vi "Get DI param from PGserver.vi"(6 "conninfo":T1={"host"="localhost", "port"="5432", "client_encoding"="WIN1251", "dbname"="data", "user"="postgres", "password"=""}, 7 "KFM":string[](array[string]), 8 "error in (no error)":errorcluster, 9 "DIParamColumns":string[](array[string])=["invert", "time_const", "module_fcode_full", "control_channel_num", "ip_adress", "fcode", "fcodef", "fcode_full", "fname"], 10 "DIParamTable":string="fd_3", 11 "DI_fcode_full":string[](array[string])) -> (0 "error out":errorcluster, 2 "Names table":string[][](array[string]), 3 "DIParameters table":dbl[][](array[numeric]))   [LabVIEW 2019, in "Inputs.lvlib"]
uses:
  Inputs.lvlib
  Database/ctl/Coninfo.ctl
  Ctl/DIParamColumns.ctl
  Database/PostgreSQL2LabVIEW/libpqlv/src/PQfinish.vi
  Database/PostgreSQL2LabVIEW/libpqlv/src/PQconnectdb.vi
  Database/PostgreSQL2LabVIEW/libpqlv/src/PQerrorMessage.vi
  Database/PostgreSQL2LabVIEW/libpqlv/src/PQstatus.vi
  <vilib>/dlg_ctls.llb/Space Constant.vi
  Database/Progress.vi
  Database/PostgreSQL2LabVIEW/libpqUtility/libpqutility.lvlib
  Database/PostgreSQL.lvlib
  Database/PostgreSQL2LabVIEW/libpqUtility64/libpqutility64.lvlib
panel:
  out "PQStatus":T2(ring)
  # "fcode_full"
  # "fname"
  # "time_const"
  # "ip_adress"
  # "fcodef"
  # "control_channel_num"
  # "instrument_offset"
  # "module_num"
  # "fcode"
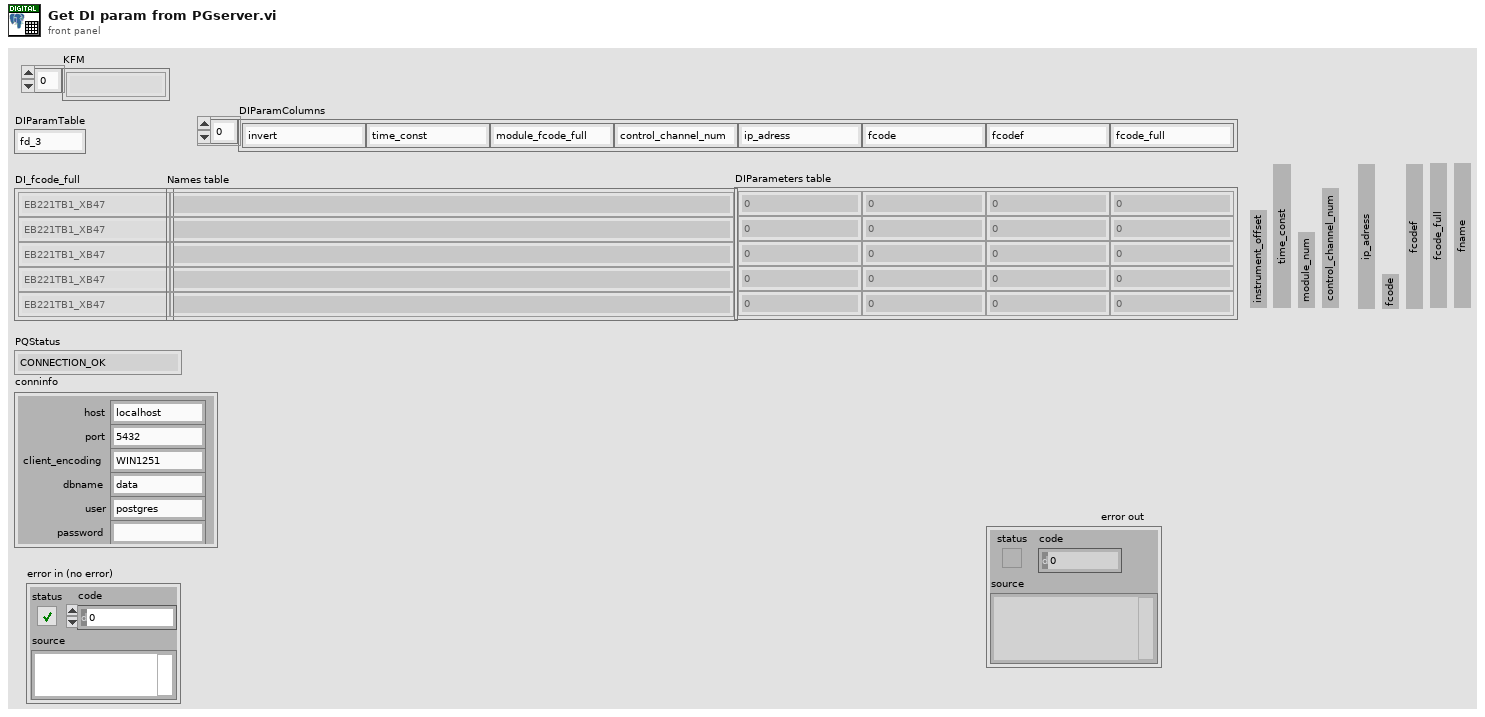
[diagram p1: front panel]
types:
  T1 = typedef "PostgreSQL.lvlib/Coninfo.ctl" = cluster{"host":string, "port":string, "client_encoding":string, "dbname":string, "user":string, "password":string}
  T2 = enum16{"CONNECTION_OK", "CONNECTION_BAD", "CONNECTION_STARTED", "CONNECTION_MADE", "CONNECTION_AWAITING_RESPONSE", "CONNECTION_AUTH_OK", "CONNECTION_SETENV", "CONNECTION_SSL_STARTUP", "CONNECTION_NEEDED"}
  T3 = typedef "Inputs.lvlib/DIParamColumns.ctl" = enum16{"invert", "time_const", "module_fcode_full", "control_channel_num", "ip_adress", "fcode", "fcodef", "fcode_full", "fname"}
  T4 = enum32{"CONNECTION_OK", "CONNECTION_BAD", "CONNECTION_STARTED", "CONNECTION_MADE", "CONNECTION_AWAITING_RESPONSE", "CONNECTION_AUTH_OK", "CONNECTION_SETENV", "CONNECTION_SSL_STARTUP", "CONNECTION_NEEDED"}
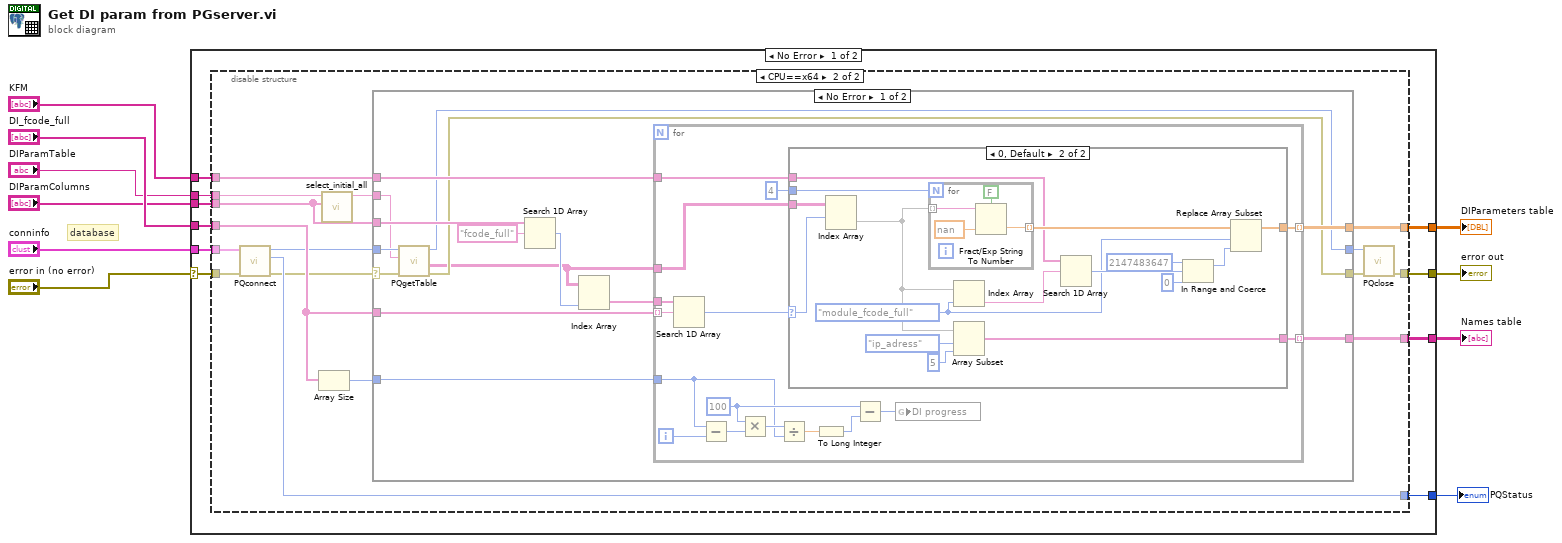
[diagram p0: block diagram]
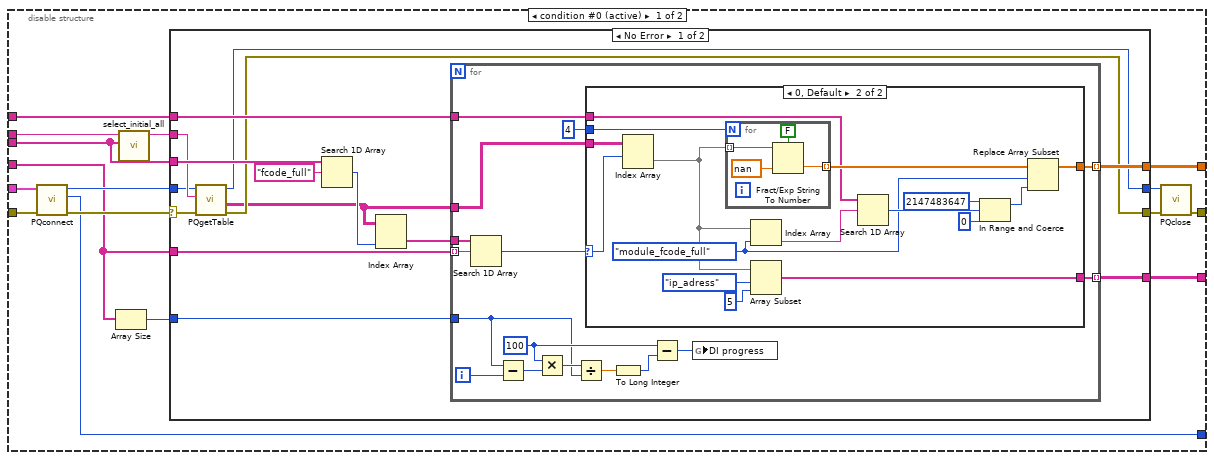
[diagram p2: hidden frame]
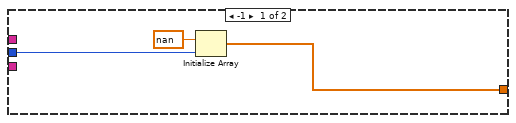
[diagram p3: hidden frame]
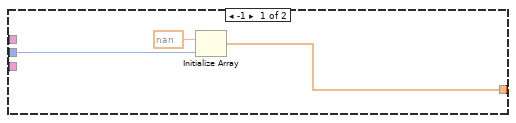
[diagram p5: hidden frame]
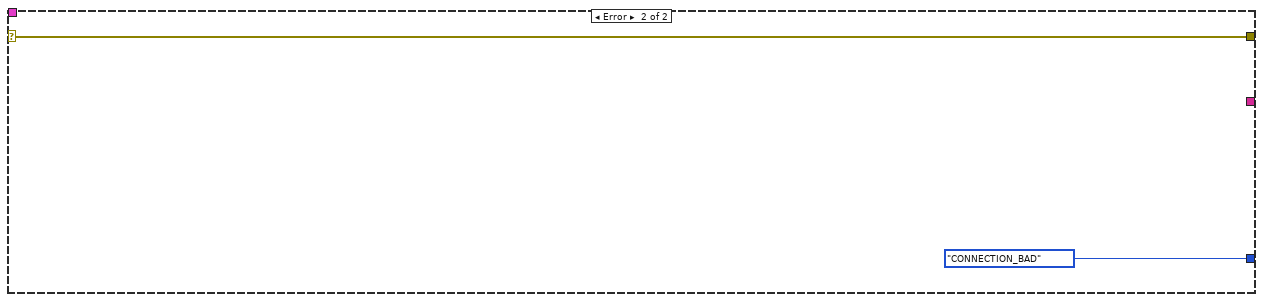
[diagram p7: hidden frame]
diagram:
  # "database"
  n1 = case shown="No Error" "error in (no error)" {
    selector: "error in (no error)" -> [w15 w166]
    tunnel: "DI_fcode_full" -> [w17 _]
    tunnel: "DIParamTable" -> [w19 _]
    tunnel: "DIParamColumns" -> [w18 _]
    tunnel: [w14 _] -> w7
    tunnel: [w13 w166] -> w6
    tunnel: [w12 _] -> w5
    tunnel: "conninfo" -> [w16 _]
    tunnel: "KFM" -> [w20 _]
    tunnel: [w11 T4."CONNECTION_BAD" ("PQStatus")] -> w1
    frame No Error {
      n2 = disable-structure shown="CPU==x64" {
        disable-tunnel: [w24 w99] -> w13
        disable-tunnel: [w29 w101] -> w14
        disable-tunnel: [w28 w102] -> w12
        disable-tunnel: w18 -> [w21 w104]
        disable-tunnel: w16 -> [w33 w97]
        disable-tunnel: w19 -> [w23 w105]
        disable-tunnel: w17 -> [w30 w103]
        disable-tunnel: w15 -> [w32 w96]
        disable-tunnel: w20 -> [w31 w106]
        disable-tunnel: [w27 w94] -> w11
        frame condition #0 (active) {
          n3 = call "PQconnect.vi"("error in (no error)"=w32, "conninfo"=w33) -> ("error out"=w36:errorcluster, "PQStatus"=w27:T4, "conn"=w35:u32)  [unwired: 7 in]
          n4 = Array Size(array=w30) -> (size(s)=w34:i32)
          n5 = call "select_initial_all.vi"("Column table"=w21, "table"=w23) -> ("parameters"=w22:string)  [unwired: 8 in, 1 out]
          n6 = case shown="No Error" w36 {
            selector: w36 -> [w43 w92]
            tunnel: w30 -> [w37 _]
            tunnel: [w51 _] -> w29
            tunnel: [w50 _] -> w28
            tunnel: w34 -> [w49 _]
            tunnel: w35 -> [w41 w91]
            tunnel: w22 -> [w42 _]
            tunnel: w31 -> [w48 _]
            tunnel: [w40 w92] -> w25
            tunnel: [w39 w91] -> w26
            tunnel: w21 -> [w44 _]
            frame No Error {
              n7 = call "PQgetTable.vi"("error in"=w43, "query"=w42, "conn"=w41) -> ("error out"=w40:errorcluster, "Data"=w38:string[][], "conn_out"=w39:u32)  [unwired: 4 in, 2 out]
              n8 = Search 1D Array(1D array=w44, element="fcode_full" ("table")) -> (index of element=w46:i32)  [unwired: 1 in]
              n9 = Index Array(array=w38, index (col)=w46) -> (element=w45:string[])  [unwired: 1 in]
              n10 = for {
                tunnel: [w67] -> w50 mode=indexing
                tunnel: [w66] -> w51 mode=indexing
                tunnel: w49 -> [w58]
                tunnel: w48 -> [w56]
                tunnel: w45 -> [w55]
                tunnel: w38 -> [w54]
                tunnel: w37 -> [w53] mode=indexing
                i -> [w59]
                w63 = 100 ("y")
                n11 = Search 1D Array(1D array=w55, element=w53) -> (index of element=w52:i32)  [unwired: 1 in]
                n12 = Subtract(x=w58, y=w59) -> (x-y=w62:i32)
                n13 = Multiply(x=w63, y=w62) -> (x*y=w65:i32)
                n14 = Divide(x=w65, y=w58) -> (x/y=w61:dbl)
                n15 = case shown="0, Default" w52 {
                  selector: w52 -> [_ w73]
                  tunnel: [w69 w78] -> w66
                  tunnel: 4 ("y") -> [w68 w83]
                  tunnel: w54 -> [_ w82]
                  tunnel: [_ w84] -> w67
                  tunnel: w56 -> [_ w80]
                  frame -1 {
                    n16 = Initialize Array(nan, w68) -> (w69:dbl[])
                  }
                  frame 0, Default {
                    w72 = DIParamColumns."module_fcode_full" ("DIParamColumns")
                    n17 = Index Array(array=w82, index (row)=w73) -> (element=w81:string[])  [unwired: 1 in]
                    n18 = for {
                      N: w83 -> [_]
                      tunnel: w81 -> [w89] mode=indexing
                      tunnel: [w88] -> w86 mode=indexing
                      n19 = Fract/Exp String To Number(use system decimal point (T)=FALSE, string=w89, default (0 dbl)=nan) -> (number=w88:dbl)  [unwired: 1 in, 1 out]
                    }
                    n20 = Index Array(array=w81, index=w72) -> (element=w79:string)
                    n21 = Array Subset(array=w81, index=DIParamColumns."ip_adress" ("DIParamColumns"), length=5) -> (w84:string[])
                    n22 = Search 1D Array(1D array=w80, element=w79) -> (index of element=w77:i32)  [unwired: 1 in]
                    n23 = In Range and Coerce(upper limit=2147483647, x=w77, lower limit=0) -> (coerced(x)=w74:i32)  [unwired: 1 out]
                    n24 = Replace Array Subset(array=w86, new element=w74, index=w72) -> (w78:dbl[])
                  }
                }
                n25 = To Long Integer(number=w61) -> (32bit integer=w60:i32)
                n26 = Subtract(x=w63, y=w60) -> (x-y=w64:i32)
                n27 = global write "Progress.vi" "DI progress"(w64) -> ()
              }
            }
            frame Error {
            }
          }
          n28 = call "PQclose.vi"("error in (no error)"=w25, "conn"=w26) -> ("error out"=w24:errorcluster)  [unwired: 9 in]
        }
        frame condition #1 {
          n29 = call "PQconnect.vi"("error in (no error)"=w96, "conninfo"=w97) -> ("error out"=w93:errorcluster, "PQStatus"=w94:T4, "conn"=w95:u64)  [unwired: 7 in]
          n30 = Array Size(array=w103) -> (size(s)=w108:i32)
          n31 = call "select_initial_all.vi"("Column table"=w104, "table"=w105) -> ("parameters"=w107:string)  [unwired: 8 in, 1 out]
          n32 = case shown="No Error" w93 {
            selector: w93 -> [w114 w164]
            tunnel: w103 -> [w115 _]
            tunnel: [w123 _] -> w101
            tunnel: [w122 _] -> w102
            tunnel: w108 -> [w121 _]
            tunnel: w95 -> [w111 w163]
            tunnel: w107 -> [w109 _]
            tunnel: w106 -> [w120 _]
            tunnel: [w113 w164] -> w100
            tunnel: [w110 w163] -> w98
            tunnel: w104 -> [w116 _]
            frame No Error {
              n33 = call "PQgetTable.vi"("error in"=w114, "query"=w109, "conn"=w111) -> ("error out"=w113:errorcluster, "Data"=w112:string[][], "conn_out"=w110:u64)  [unwired: 4 in, 2 out]
              n34 = Search 1D Array(1D array=w116, element="fcode_full" ("table")) -> (index of element=w118:i32)  [unwired: 1 in]
              n35 = Index Array(array=w112, index (col)=w118) -> (element=w117:string[])  [unwired: 1 in]
              n36 = for {
                tunnel: [w139] -> w122 mode=indexing
                tunnel: [w138] -> w123 mode=indexing
                tunnel: w121 -> [w130]
                tunnel: w120 -> [w128]
                tunnel: w117 -> [w127]
                tunnel: w112 -> [w126]
                tunnel: w115 -> [w125] mode=indexing
                i -> [w131]
                w135 = 100 ("y")
                n37 = Search 1D Array(1D array=w127, element=w125) -> (index of element=w124:i32)  [unwired: 1 in]
                n38 = Subtract(x=w130, y=w131) -> (x-y=w134:i32)
                n39 = Multiply(x=w135, y=w134) -> (x*y=w137:i32)
                n40 = Divide(x=w137, y=w130) -> (x/y=w133:dbl)
                n41 = case shown="0, Default" w124 {
                  selector: w124 -> [_ w145]
                  tunnel: [w141 w150] -> w138
                  tunnel: 4 ("y") -> [w140 w155]
                  tunnel: w126 -> [_ w154]
                  tunnel: [_ w156] -> w139
                  tunnel: w128 -> [_ w152]
                  frame -1 {
                    n42 = Initialize Array(nan, w140) -> (w141:dbl[])
                  }
                  frame 0, Default {
                    w143 = DIParamColumns."module_fcode_full" ("DIParamColumns")
                    n43 = Index Array(array=w154, index (row)=w145) -> (element=w153:string[])  [unwired: 1 in]
                    n44 = for {
                      N: w155 -> [_]
                      tunnel: w153 -> [w161] mode=indexing
                      tunnel: [w160] -> w158 mode=indexing
                      n45 = Fract/Exp String To Number(use system decimal point (T)=FALSE, string=w161, default (0 dbl)=nan) -> (number=w160:dbl)  [unwired: 1 in, 1 out]
                    }
                    n46 = Index Array(array=w153, index=w143) -> (element=w151:string)
                    n47 = Array Subset(array=w153, index=DIParamColumns."ip_adress" ("DIParamColumns"), length=5) -> (w156:string[])
                    n48 = Search 1D Array(1D array=w152, element=w151) -> (index of element=w149:i32)  [unwired: 1 in]
                    n49 = In Range and Coerce(upper limit=2147483647, x=w149, lower limit=0) -> (coerced(x)=w146:i32)  [unwired: 1 out]
                    n50 = Replace Array Subset(array=w158, new element=w146, index=w143) -> (w150:dbl[])
                  }
                }
                n51 = To Long Integer(number=w133) -> (32bit integer=w132:i32)
                n52 = Subtract(x=w135, y=w132) -> (x-y=w136:i32)
                n53 = global write "Progress.vi" "DI progress"(w136) -> ()
              }
            }
            frame Error {
            }
          }
          n54 = call "PQclose.vi"("error in (no error)"=w100, "conn"=w98) -> ("error out"=w99:errorcluster)  [unwired: 9 in]
        }
      }
    }
    frame Error {
    }
  }
  "error out" <- w6
  "DIParameters table" <- w7
  "Names table" <- w5
  "PQStatus" <- w1
